vi "Set Slew.vi"(7 "Output Channel":T1, 8 "error in (no error)":errorcluster, 10 "Slew (V/s)":dbl, 11 "VISA resource name":refnum<visa-resource-name>) -> (0 "error out":errorcluster, 3 "VISA Refnum out":refnum<visa-resource-name>)   [LabVIEW 2016, in "RP100.lvclass"]
uses:
  RP100.lvclass
  Typedefs/Output Channel--Enum.ctl
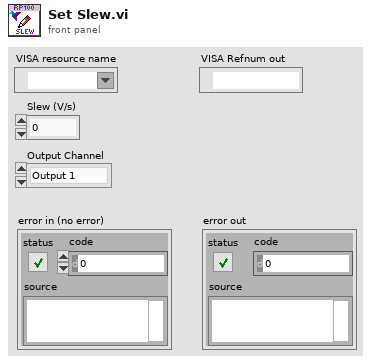
[diagram p1: front panel]
types:
  T1 = typedef "RP100.lvclass/Output Channel--Enum.ctl" = enum16{"Output 1", "Output 2"}
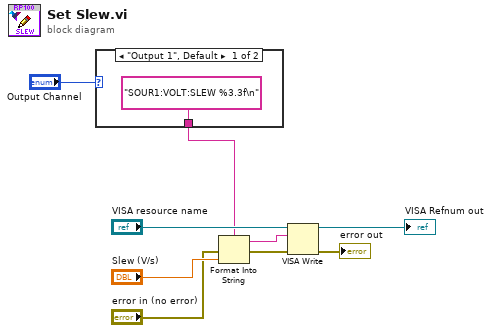
[diagram p0: block diagram]
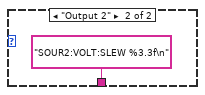
[diagram p2: hidden frame]
diagram:
  n1 = case shown="\"Output 1\", Default" "Output Channel" {
    tunnel: ["SOUR1:VOLT:SLEW %3.3f\n" ("format string") "SOUR2:VOLT:SLEW %3.3f\n" ("format string")] -> w1
    frame "Output 1", Default {
    }
    frame "Output 2" {
    }
  }
  n2 = Format Into String(format string=w1, error in="error in (no error)", "Slew (V/s)") -> (resulting string=w6:string, error out=w3:errorcluster)  [unwired: 1 in]
  n3 = VISA Write(VISA resource name="VISA resource name", write buffer=w6, error in (no error)=w3) -> (VISA resource name out=→"VISA Refnum out":refnum<visa-resource-name>, error out=→"error out":errorcluster)  [unwired: 1 out]
